vi "Manipulator PWM-y.vi"(8 "output cluster":T2, 11 "axis info":T1) -> (1 "wyj pwm manip.":T3)   [LabVIEW 2015]
uses:
  wyj manip.ctl
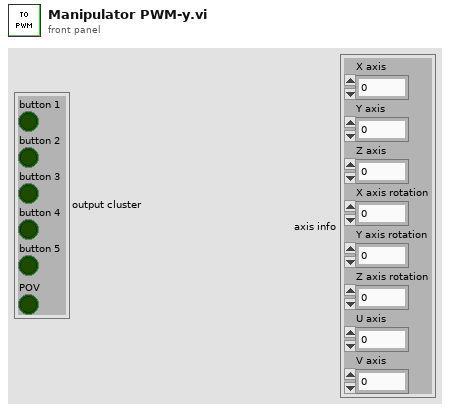
[diagram p1: front panel]
types:
  T1 = cluster{"X axis":i32, "Y axis":i32, "Z axis":i32, "X axis rotation":i32, "Y axis rotation":i32, "Z axis rotation":i32, "U axis":i32, "V axis":i32}
  T2 = typedef "wyj manip.ctl" = cluster{"button 1":bool, "button 2":bool, "button 3":bool, "button 4":bool, "button 5":bool, "POV":bool}
  T3 = cluster{"pwm 1":i16, "pwm 2":i16, "pwm 3":i16, "pwm 4":i16, "pwm 5":i16, "pwm 6":i16, "pwm 7":i16}
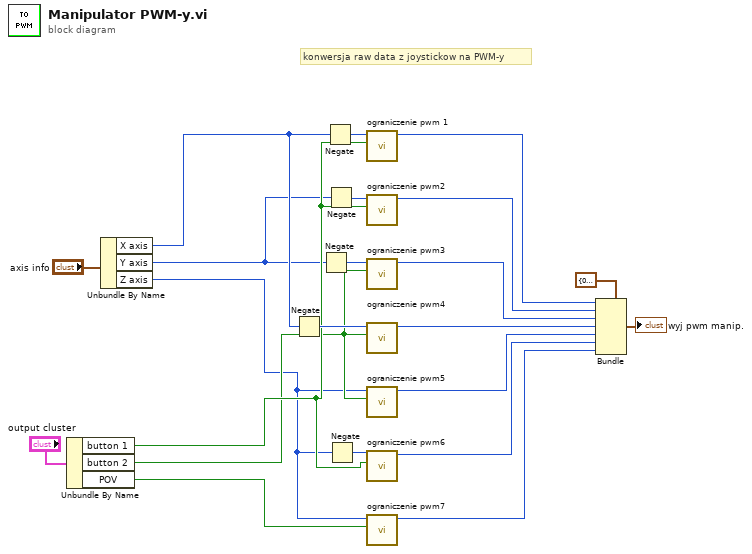
[diagram p0: block diagram]
diagram:
  # "konwersja raw data z joystickow na PWM-y"
  n1 = Unbundle By Name("output cluster") -> ("button 1"=w7:bool, "button 2"=w6:bool, "POV"=w5:bool)
  n2 = Unbundle By Name("axis info") -> ("X axis"=w3:i32, "Y axis"=w2:i32, "Z axis"=w1:i32)
  n3 = Negate(x=w3) -> (-x=w18:i32)
  n4 = Negate(x=w2) -> (-x=w19:i32)
  n5 = Negate(x=w3) -> (-x=w21:i32)
  n6 = Negate(x=w2) -> (-x=w20:i32)
  n7 = Negate(x=w1) -> (-x=w22:i32)
  n8 = call "ograniczenie pwm 1.vi"("button 1"=w7, "X axis"=w21) -> ("y"=w16:i16)  [unwired: 9 in]
  n9 = call "ograniczenie pwm2.vi"("button 1"=w7, "X axis"=w20) -> ("y"=w15:i16)  [unwired: 9 in]
  n10 = call "ograniczenie pwm3.vi"("button 1"=w6, "X axis"=w19) -> ("y"=w14:i16)  [unwired: 9 in]
  n11 = call "ograniczenie pwm4.vi"("button 1"=w6, "X axis"=w18) -> ("y"=w13:i16)  [unwired: 9 in]
  n12 = call "ograniczenie pwm5.vi"("button 1"=w6, "X axis"=w1) -> ("y"=w12:i16)  [unwired: 9 in]
  n13 = call "ograniczenie pwm6.vi"("button 1"=w7, "X axis"=w22) -> ("y"=w11:i16)  [unwired: 9 in]
  n14 = call "ograniczenie pwm7.vi"("button 1"=w5, "X axis"=w1) -> ("y"=w10:i16)  [unwired: 9 in]
  n15 = Bundle(cluster=T3 {"pwm 1"=0, "pwm 2"=0, "pwm 3"=0, "pwm 4"=0, "pwm 5"=0, "pwm 6"=0, "pwm 7"=0} ("output cluster"), "pwm 1"=w16, "pwm 2"=w15, "pwm 3"=w14, "pwm 4"=w13, "pwm 5"=w12, "pwm 6"=w11, "pwm 7"=w10) -> (→"wyj pwm manip.":T3)
